vi "Indentify-Consequent.vi"() -> ()   [LabVIEW 2019]
panel:
  out "對應顏色":enum16{"黃", "紅", "綠", "藍", "黑", "µL"}(ring)
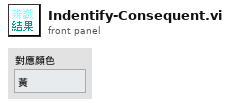
[diagram p1: front panel]
diagram:
